vi "LDA_Maths_check.vi"(0 "B1 Close P11":dbl[](array[numeric])=[2570.8702, 433.495, 303.3539], 1 "Use Specification Beam Half-Angle":bool=TRUE, 5 "B1 Far P12":dbl[](array[numeric])=[2646.4891, 432.64, 306.6406], 7 "B2 Close P22":dbl[](array[numeric]), 9 "B2 Far P21":dbl[](array[numeric])=[2643.8249, 436.46, 319.8555], 11 "Use Green Beams (True) or Blue Beams (False)":bool, 12 "Beam Half-Angle (deg)":dbl=4.572782629722086 format="%#_9g", 13 "Using 45 Degree Mirror?":bool) -> (4 "Beam Data":T1={"Vg1 (Green 1 dir. vect.)"=[-0.9913846154927373, -0.08722653267640797, -0.09771425771896834], "Vg2  (Green 2 dir. vect.)"=[-0.987756229722306, 0.06610682889995216, -0.1413064677131501], "Vb1 (Blue 1 dir. vect.)"=[-0.9989930425665134, 0.011295311772511737, -0.04342023532481111], "Vb2 (Blue 1 dir. vect.)"=[-0.9801478026485297, -0.032415015548967537, -0.19560049010730732], "Porb (Orb XYZ posn. forced coplanar)"=[2558.4254936976226, 433.635708525098, 302.8130032638134], "Porb (Orb XYZ posn. - allow skew)"=[2558.425493697624, 433.635708525098, 302.8130032638134], "Orb posn. uncertainty, +/- dx, dy, dz"=[6.821210263296962e-13, 0.0, 0.0], "Vp (Actual Probe dir. vect)"=[-0.9927304194336236, -0.010593572680289348, -0.11989199535001965], "Yaw (deg)"=179.38861149501568, "Pitch (deg)"=-6.885869367545546, "In-Plane Roll (deg)"=15.984421506271559, "Beam Half Angle (deg)"=4.572782629722086, "B1 Close P11"=[2570.8702, 433.495, 303.3539], "B1 Far P12"=[2646.4891, 432.64, 306.6406], "B2 Close P22"=[nan, nan, nan], "B2 Far P21"=[2643.8249, 436.46, 319.8555], "Projected Roll (deg)"=15.87029035209838, "Green Velocity Vector"=[-0.022755515757454235, -0.9616341663360687, 0.273389679098803], "Blue Velocity Vector"=[0.1181884124343585, -0.2741304549899585, -0.9544024270784544], "Probe is facing...."="Upstream (YZ)", "Calculation Method"=""} {"Vp (Actual Probe dir. vect)" format="%#_6f"; "Vg2  (Green 2 dir. vect.)" format="%#_6f"; "Vg1 (Green 1 dir. vect.)" format="%#_6f"})   [LabVIEW 2011]
uses:
  Controls/LDA_Beam_Cluster.ctl
  <vilib>/Analysis/baseanly.llb/Unit Vector (DBL).vi
  <vilib>/Analysis/baseanly.llb/Real Dot Product.vi
  <vilib>/Analysis/NI_AALBase.lvlib
panel:
  # "Please note angle conventions:\nClockwise positive looking into the axis of rotation"
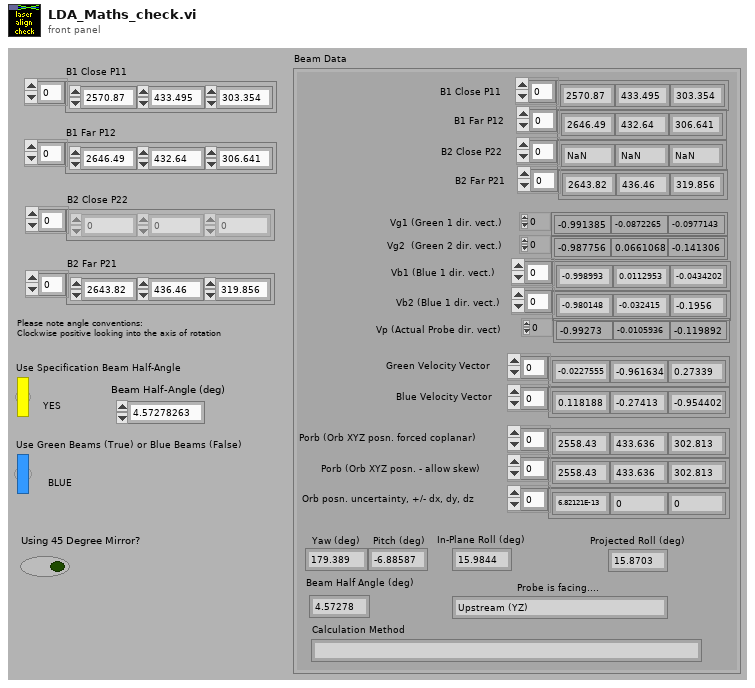
[diagram p1: front panel]
types:
  T1 = typedef "LDA_Beam_Cluster.ctl" = cluster{"Vg1 (Green 1 dir. vect.)":dbl[], "Vg2  (Green 2 dir. vect.)":dbl[], "Vb1 (Blue 1 dir. vect.)":dbl[], "Vb2 (Blue 1 dir. vect.)":dbl[], "Porb (Orb XYZ posn. forced coplanar)":dbl[], "Porb (Orb XYZ posn. - allow skew)":dbl[], "Orb posn. uncertainty, +/- dx, dy, dz":dbl[], "Vp (Actual Probe dir. vect)":dbl[], "Yaw (deg)":dbl, "Pitch (deg)":dbl, "In-Plane Roll (deg)":dbl, "Beam Half Angle (deg)":dbl, "B1 Close P11":dbl[], "B1 Far P12":dbl[], "B2 Close P22":dbl[], "B2 Far P21":dbl[], "Projected Roll (deg)":dbl, "Green Velocity Vector":dbl[], "Blue Velocity Vector":dbl[], "Probe is facing....":string, "Calculation Method":string}
  T2 = cluster{"Unit Vector[0]":dbl, "Unit Vector[1]":dbl, "Unit Vector[2]":dbl}
  T3 = cluster{"input variable":dbl, "input variable":dbl, "input variable":dbl}
  T4 = cluster{"input variable":dbl, dbl, "input variable":dbl}
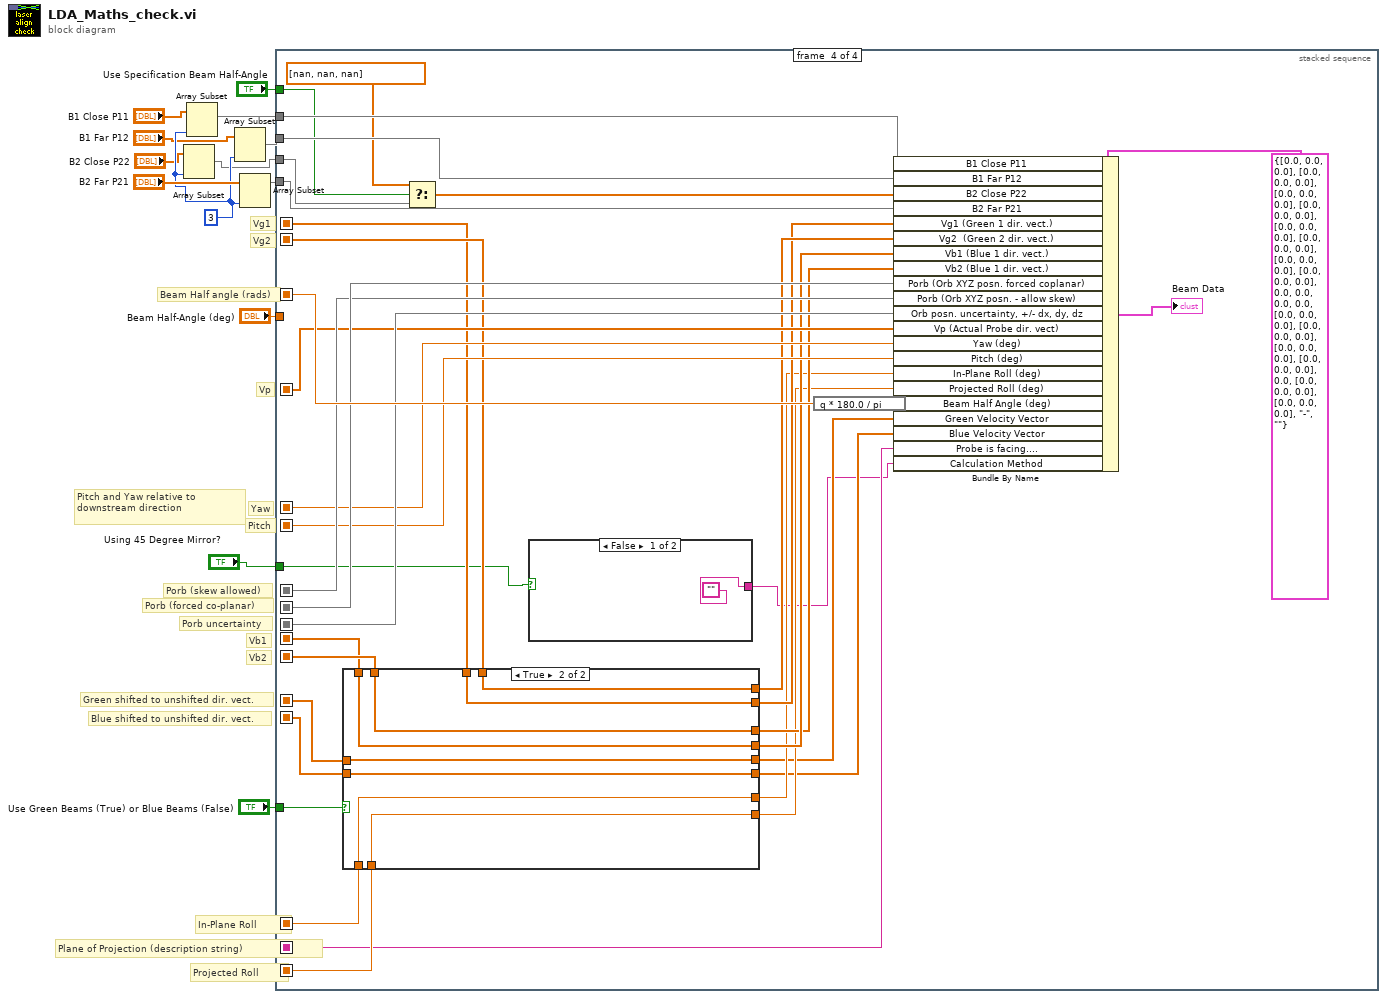
[diagram p0: block diagram]
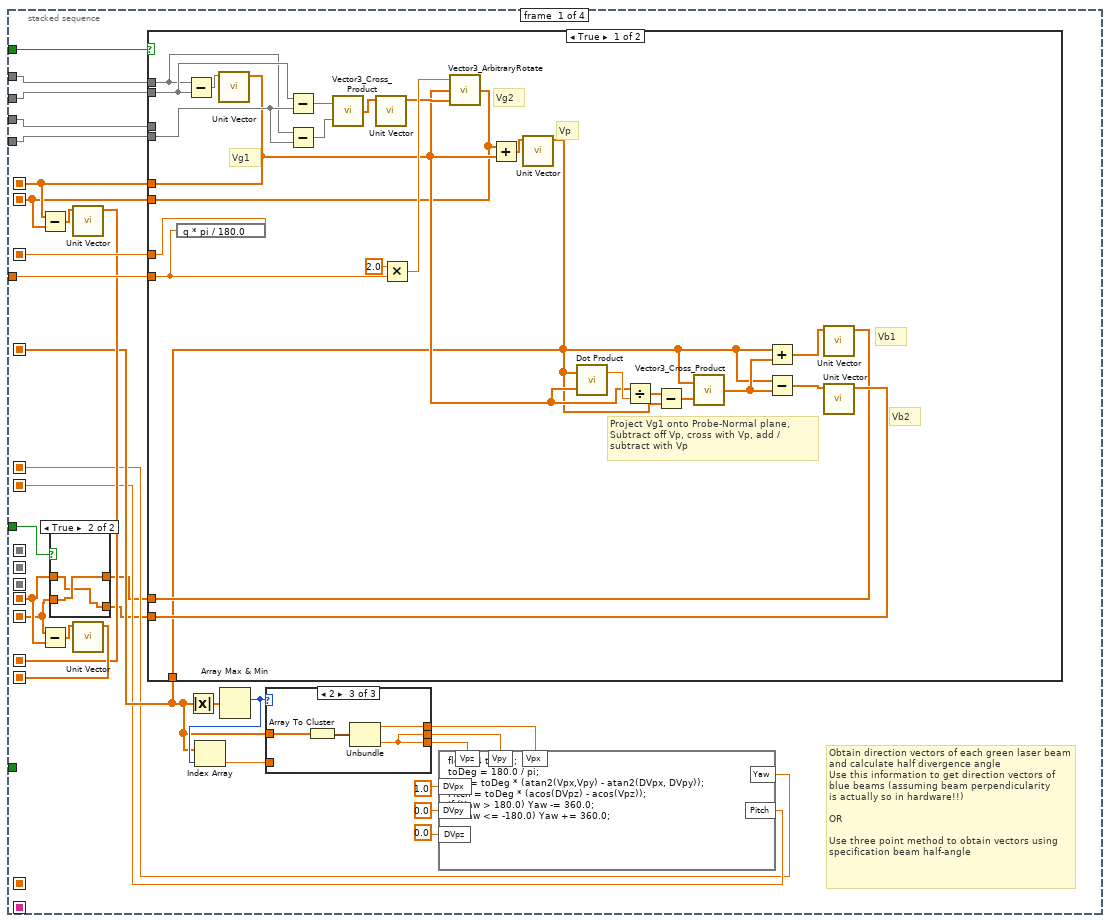
[diagram p2: hidden frame]
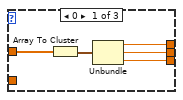
[diagram p4: hidden frame]
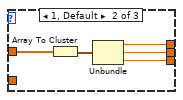
[diagram p5: hidden frame]
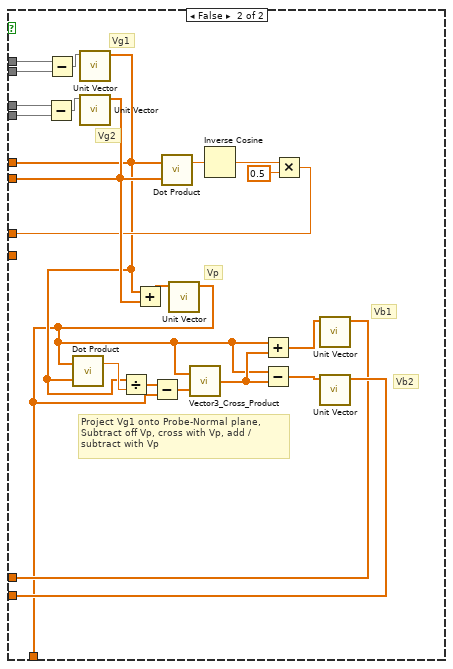
[diagram p6: hidden frame]
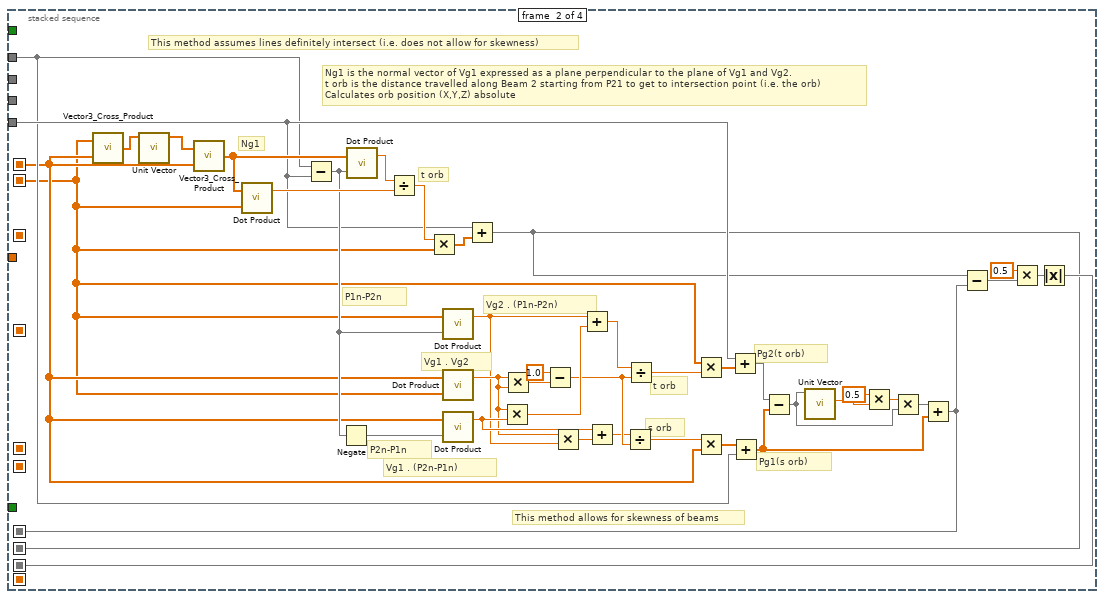
[diagram p7: hidden frame]
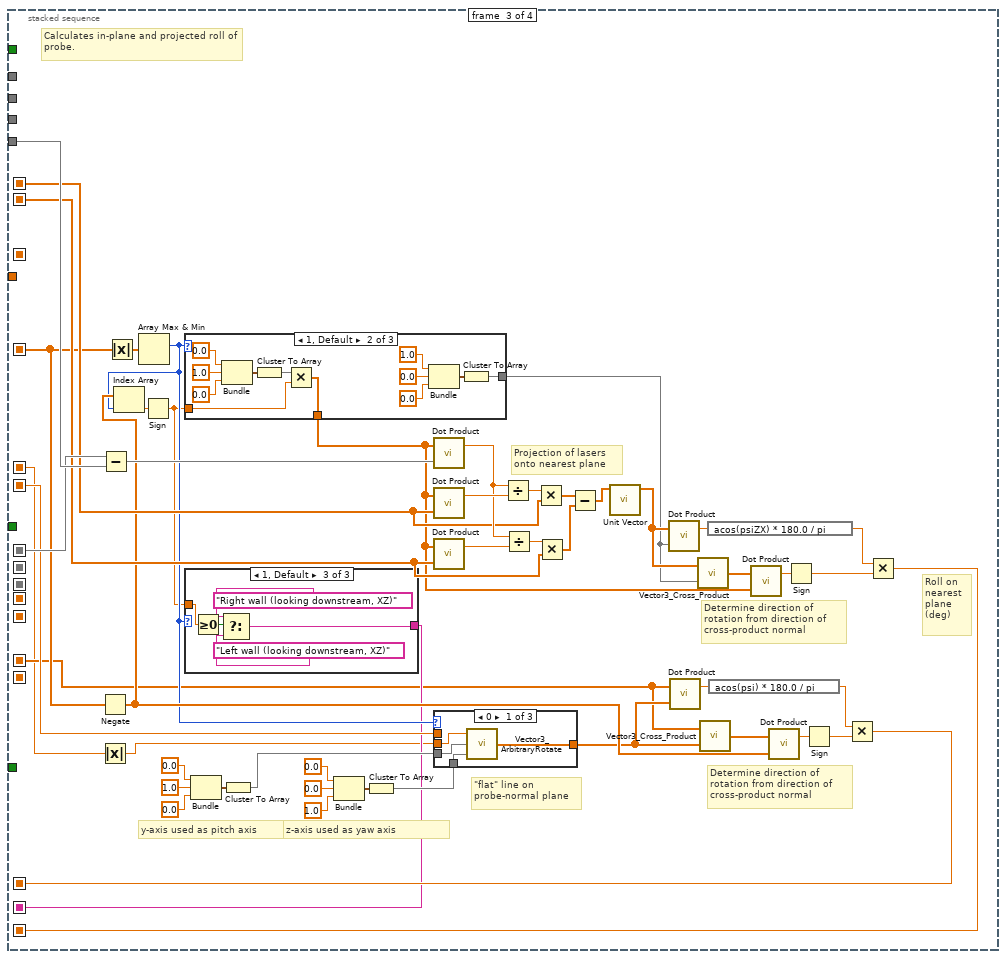
[diagram p8: hidden frame]
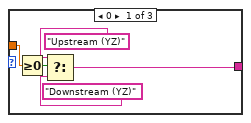
[diagram p9: hidden frame]
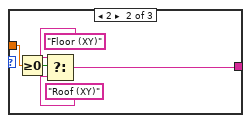
[diagram p10: hidden frame]
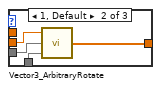
[diagram p11: hidden frame]
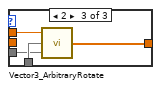
[diagram p12: hidden frame]
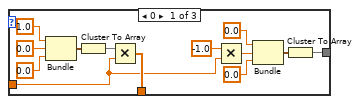
[diagram p13: hidden frame]
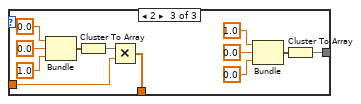
[diagram p14: hidden frame]
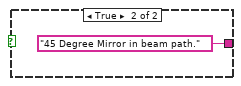
[diagram p15: hidden frame]
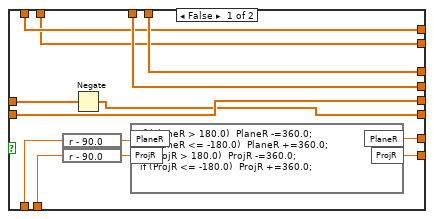
[diagram p16: hidden frame]
diagram:
  w5 = 3 ("length")
  # "Plane of Projection (description string)"
  # "Blue shifted to unshifted dir. vect."
  # "Green shifted to unshifted dir. vect."
  # "Projected Roll"
  # "Porb (forced co-planar)"
  # "Porb uncertainty"
  # "In-Plane Roll"
  # "Pitch"
  # "Yaw"
  # "Vb2"
  # "Vb1"
  # "Pitch and Yaw relative to\ndownstream direction"
  # "Vp"
  # "Porb (skew allowed)"
  # "Beam Half angle (rads)"
  # "Vg2"
  # "Vg1"
  n1 = Array Subset(array="B2 Close P22", length=w5) -> (w3:dbl[])  [unwired: 1 in]
  n2 = Array Subset(array="B1 Close P11", length=w5) -> (w6:dbl[])  [unwired: 1 in]
  n3 = Array Subset(array="B1 Far P12", length=w5) -> (w8:dbl[])  [unwired: 1 in]
  n4 = Array Subset(array="B2 Far P21", length=w5) -> (w9:dbl[])  [unwired: 1 in]
  n5 = stacked-sequence {
    seq-local: [w36 _ _ _] -> [_ w109 w171 w281]
    seq-local: [w35 _ _ _] -> [_ w108 w170 w282]
    seq-local: [w42 _ _ _] -> [_ _ _ w297]
    seq-local: [_ w112 _ _] -> [_ _ w177 w295]
    seq-local: [w24 _ _ _] -> [_ _ w162 w293]
    seq-local: [w17 _ _ _] -> [_ _ _ w279]
    seq-local: [w15 _ _ _] -> [_ _ _ w280]
    seq-local: [w19 _ _ _] -> [_ _ w150 w292]
    seq-local: [w20 _ _ _] -> [_ _ w176 w291]
    seq-local: [_ _ w179 _] -> [_ _ _ w273]
    seq-local: [_ w111 _ _] -> [_ _ _ w294]
    seq-local: [_ w110 _ _] -> [_ _ _ w296]
    seq-local: [_ _ w154 _] -> [_ _ _ w271]
    seq-local: [w31 _ _ _] -> [_ _ w151 w268]
    seq-local: [w33 _ _ _] -> [_ _ _ w269]
    seq-local: [_ _ w152 _] -> [_ _ _ w265]
    tunnel: w6 -> [w39 w123 _ w288]
    tunnel: w8 -> [w41 _ _ w289]
    tunnel: w3 -> [w43 _ _ w285]
    tunnel: w9 -> [w40 w128 w178 w290]
    tunnel: "Beam Half-Angle (deg)" -> [w38 _ _ _]
    tunnel: "Use Specification Beam Half-Angle" -> [w37 _ _ w286]
    tunnel: "Use Green Beams (True) or Blue Beams (False)" -> [_ _ _ w278]
    tunnel: "Using 45 Degree Mirror?" -> [w18 _ _ w263]
    frame #0 {
      # "Obtain direction vectors of each green laser beam and calculate half divergence angle\nUse this information to get direction vectors of blue beams (assuming beam perpendicularity\nis actually so in hardware!!)\n\nOR\n\nUse three point method to obtain vectors using specification beam half-angle"
      n6 = case shown="True" w37 {
        tunnel: w43 -> [_ w105]
        tunnel: [w67 w102] -> w35
        tunnel: [w64 w98] -> w42
        tunnel: [w66 w93] -> w14
        tunnel: w41 -> [w84 w92]
        tunnel: w40 -> [w83 w91]
        tunnel: w39 -> [w82 w90]
        tunnel: w38 -> [w63 _]
        tunnel: [w65 w89] -> w16
        tunnel: [w68 w87] -> w36
        tunnel: [w62 w86] -> w24
        frame True {
          # "Vg1"
          # "Vb2"
          # "Vb1"
          # "Vp"
          # "Vg2"
          # "Project Vg1 onto Probe-Normal plane, Subtract off Vp, cross with Vp, add / subtract with Vp"
          n7 = expression code="q * pi / 180.0"(w63) -> (w64:dbl)
          n8 = Subtract(x=w82, y=w84) -> (x-y=w85:dbl[])
          n9 = call-poly <vilib>:"Unit Vector.vi"("Input Vector"=w85) -> ("Unit Vector"=w68:dbl[])  [unwired: 2 in, 8 out]
          n10 = Subtract(x=w84, y=w83) -> (x-y=w81:dbl[])
          n11 = Subtract(x=w82, y=w83) -> (x-y=w80:dbl[])
          n12 = call "Vector3_Cross_Product.vi"("V"=w80, "U"=w81) -> ("UxV"=w79:dbl[])
          n13 = call-poly <vilib>:"Unit Vector.vi"("Input Vector"=w79) -> ("Unit Vector"=w76:dbl[])  [unwired: 2 in, 8 out]
          n14 = Multiply(x=2.0 ("y"), y=w63) -> (x*y=w77:dbl)
          n15 = call "Vector3_ArbitraryRotate.vi"("Arbitrary Axis (as UNIT Vector3)"=w76, "Input Vector3"=w68, "Rotation angle (deg)"=w77) -> ("Output Vector3"=w67:dbl[])
          n16 = Add(x=w67, y=w68) -> (x+y=w75:dbl[])
          n17 = call-poly <vilib>:"Unit Vector.vi"("Input Vector"=w75) -> ("Unit Vector"=w62:dbl[])  [unwired: 2 in, 8 out]
          n18 = call-poly <vilib>:"Dot Product.vi"("Y Vector"=w68, "X Vector"=w62) -> ("X * Y"=w70:dbl)  [unwired: 1 out]
          n19 = Divide(x=w68, y=w70) -> (x/y=w71:dbl[])
          n20 = Subtract(x=w71, y=w62) -> (x-y=w72:dbl[])
          n21 = call "Vector3_Cross_Product.vi"("V"=w72, "U"=w62) -> ("UxV"=w73:dbl[])
          n22 = Add(x=w62, y=w73) -> (x+y=w74:dbl[])
          n23 = Subtract(x=w62, y=w73) -> (x-y=w69:dbl[])
          n24 = call-poly <vilib>:"Unit Vector.vi"("Input Vector"=w74) -> ("Unit Vector"=w65:dbl[])  [unwired: 2 in, 8 out]
          n25 = call-poly <vilib>:"Unit Vector.vi"("Input Vector"=w69) -> ("Unit Vector"=w66:dbl[])  [unwired: 2 in, 8 out]
        }
        frame False {
          # "Vg2"
          # "Vg1"
          # "Vb2"
          # "Vb1"
          # "Vp"
          # "Project Vg1 onto Probe-Normal plane, Subtract off Vp, cross with Vp, add / subtract with Vp"
          n26 = Subtract(x=w105, y=w91) -> (x-y=w106:dbl[])
          n27 = Subtract(x=w90, y=w92) -> (x-y=w107:dbl[])
          n28 = call-poly <vilib>:"Unit Vector.vi"("Input Vector"=w107) -> ("Unit Vector"=w87:dbl[])  [unwired: 2 in, 8 out]
          n29 = call-poly <vilib>:"Unit Vector.vi"("Input Vector"=w106) -> ("Unit Vector"=w102:dbl[])  [unwired: 2 in, 8 out]
          n30 = Add(x=w87, y=w102) -> (x+y=w101:dbl[])
          n31 = call-poly <vilib>:"Dot Product.vi"("Y Vector"=w102, "X Vector"=w87) -> ("X * Y"=w100:dbl)  [unwired: 1 out]
          n32 = call-poly <vilib>:"Unit Vector.vi"("Input Vector"=w101) -> ("Unit Vector"=w86:dbl[])  [unwired: 2 in, 8 out]
          n33 = call-poly <vilib>:"Dot Product.vi"("Y Vector"=w87, "X Vector"=w86) -> ("X * Y"=w97:dbl)  [unwired: 1 out]
          n34 = Divide(x=w87, y=w97) -> (x/y=w96:dbl[])
          n35 = Subtract(x=w96, y=w86) -> (x-y=w95:dbl[])
          n36 = call "Vector3_Cross_Product.vi"("V"=w95, "U"=w86) -> ("UxV"=w94:dbl[])
          n37 = Inverse Cosine(1:w100) -> (0:w104:dbl)
          n38 = Add(x=w86, y=w94) -> (x+y=w88:dbl[])
          n39 = Subtract(x=w86, y=w94) -> (x-y=w99:dbl[])
          n40 = Multiply(x=w104, y=0.5) -> (x*y=w98:dbl)
          n41 = call-poly <vilib>:"Unit Vector.vi"("Input Vector"=w88) -> ("Unit Vector"=w89:dbl[])  [unwired: 2 in, 8 out]
          n42 = call-poly <vilib>:"Unit Vector.vi"("Input Vector"=w99) -> ("Unit Vector"=w93:dbl[])  [unwired: 2 in, 8 out]
        }
      }
      n43 = Subtract(x=w36, y=w35) -> (x-y=w32:dbl[])
      n44 = case shown="True" w18 {
        tunnel: [w45 w46] -> w17
        tunnel: w16 -> [w45 w47]
        tunnel: [w44 w47] -> w15
        tunnel: w14 -> [w44 w46]
        frame False {
        }
        frame True {
        }
      }
      n45 = Subtract(x=w15, y=w17) -> (x-y=w34:dbl[])
      n46 = call-poly <vilib>:"Unit Vector.vi"("Input Vector"=w32) -> ("Unit Vector"=w31:dbl[])  [unwired: 2 in, 8 out]
      n47 = call-poly <vilib>:"Unit Vector.vi"("Input Vector"=w34) -> ("Unit Vector"=w33:dbl[])  [unwired: 2 in, 8 out]
      n48 = Absolute Value(x=w24) -> (abs(x)=w30:dbl[])
      n49 = Array Max & Min(array=w30) -> (max index (indices)=w29:i32)  [unwired: 3 out]
      n50 = Index Array(array=w24, index=w29) -> (element=w25:dbl)
      n51 = case shown="2" w29 {
        tunnel: w25 -> [_ _ _]
        tunnel: w24 -> [w51 w56 w60]
        tunnel: [w50 w53 w59] -> w21
        tunnel: [w49 w54 w59] -> w22
        tunnel: [w48 w55 w58] -> w23
        frame 0 {
          n52 = Array To Cluster(array=w51) -> (cluster=w52:T2)
          n53 = Unbundle(w52) -> ("Unit Vector[0]"=w48:dbl, "Unit Vector[1]"=w49:dbl, "Unit Vector[2]"=w50:dbl)
        }
        frame 1, Default {
          n54 = Array To Cluster(array=w56) -> (cluster=w57:T2)
          n55 = Unbundle(w57) -> ("Unit Vector[0]"=w55:dbl, "Unit Vector[1]"=w54:dbl, "Unit Vector[2]"=w53:dbl)
        }
        frame 2 {
          n56 = Array To Cluster(array=w60) -> (cluster=w61:T2)
          n57 = Unbundle(w61) -> ("Unit Vector[0]"=w58:dbl, "Unit Vector[2]"=w59:dbl)  [unwired: 1 out]
        }
      }
      n58 = formula code="float64 toDeg;\ntoDeg = 180.0 / pi;\nYaw = toDeg * (atan2(Vpx,Vpy) - atan2(DVpx, DVpy));\nPitch = toDeg * (acos(DVpz) - acos(Vpz));\nif (Yaw > 180.0) Yaw -= 360.0;\nif (Yaw <= -180.0) Yaw += 360.0;"("Vpx"=w23, "Vpy"=w22, "Vpz"=w21, "DVpx"=1.0 ("input variable"), "DVpy"=0.0 ("input variable"), "DVpz"=0.0 ("input variable")) -> ("Yaw"=w19:dbl, "Pitch"=w20:dbl)
    }
    frame #1 {
      # "Pg1(s orb)"
      # "Pg2(t orb)"
      # "s orb"
      # "t orb"
      # "Vg1 . (P2n-P1n)"
      # "Vg1 . Vg2"
      # "Vg2 . (P1n-P2n)"
      # "P2n-P1n"
      # "P1n-P2n"
      # "This method allows for skewness of beams"
      # "This method assumes lines definitely intersect (i.e. does not allow for skewness)"
      # "t orb"
      # "Ng1 is the normal vector of Vg1 expressed as a plane perpendicular to the plane of Vg1 and Vg2.\nt orb is the distance travelled along Beam 2 starting from P21 to get to intersection point (i.e. the orb)\nCalculates orb position (X,Y,Z) absolute"
      # "Ng1"
      n59 = call "Vector3_Cross_Product.vi"("V"=w109, "U"=w108) -> ("UxV"=w143:dbl[])
      n60 = call-poly <vilib>:"Unit Vector.vi"("Input Vector"=w143) -> ("Unit Vector"=w142:dbl[])  [unwired: 2 in, 8 out]
      n61 = call "Vector3_Cross_Product.vi"("V"=w109, "U"=w142) -> ("UxV"=w141:dbl[])
      n62 = call-poly <vilib>:"Dot Product.vi"("Y Vector"=w108, "X Vector"=w141) -> ("X * Y"=w146:dbl)  [unwired: 1 out]
      n63 = Subtract(x=w123, y=w128) -> (x-y=w140:dbl[])
      n64 = Negate(x=w140) -> (-x=w139:dbl[])
      n65 = call-poly <vilib>:"Dot Product.vi"("Y Vector"=w140, "X Vector"=w141) -> ("X * Y"=w147:dbl)  [unwired: 1 out]
      n66 = Divide(x=w147, y=w146) -> (x/y=w145:dbl)
      n67 = Multiply(x=w145, y=w108) -> (x*y=w144:dbl[])
      n68 = call-poly <vilib>:"Dot Product.vi"("Y Vector"=w140, "X Vector"=w108) -> ("X * Y"=w132:dbl)  [unwired: 1 out]
      n69 = call-poly <vilib>:"Dot Product.vi"("Y Vector"=w108, "X Vector"=w109) -> ("X * Y"=w133:dbl)  [unwired: 1 out]
      n70 = call-poly <vilib>:"Dot Product.vi"("Y Vector"=w139, "X Vector"=w109) -> ("X * Y"=w134:dbl)  [unwired: 1 out]
      n71 = Add(x=w128, y=w144) -> (x+y=w110:dbl[])
      n72 = Multiply(x=w133, y=w134) -> (x*y=w136:dbl)
      n73 = Multiply(x=w133, y=w133) -> (x*y=w137:dbl)
      n74 = Subtract(x=1.0, y=w137) -> (x-y=w130:dbl)
      n75 = Multiply(x=w133, y=w132) -> (x*y=w131:dbl)
      n76 = Add(x=w132, y=w136) -> (x+y=w135:dbl)
      n77 = Add(x=w134, y=w131) -> (x+y=w129:dbl)
      n78 = Divide(x=w129, y=w130) -> (x/y=w125:dbl)
      n79 = Divide(x=w135, y=w130) -> (x/y=w127:dbl)
      n80 = Multiply(x=w108, y=w127) -> (x*y=w126:dbl[])
      n81 = Multiply(x=w125, y=w109) -> (x*y=w124:dbl[])
      n82 = Add(x=w128, y=w126) -> (x+y=w122:dbl[])
      n83 = Add(x=w124, y=w123) -> (x+y=w116:dbl[])
      n84 = Subtract(x=w122, y=w116) -> (x-y=w118:dbl[])
      n85 = call-poly <vilib>:"Unit Vector.vi"("Input Vector"=w118) -> ("norm"=w120:dbl)  [unwired: 2 in, 8 out]
      n86 = Multiply(x=0.5, y=w120) -> (x*y=w119:dbl)
      n87 = Multiply(x=w119, y=w118) -> (x*y=w117:dbl[])
      n88 = Add(x=w117, y=w116) -> (x+y=w112:dbl[])
      n89 = Subtract(x=w110, y=w112) -> (x-y=w114:dbl[])
      n90 = Multiply(x=0.5, y=w114) -> (x*y=w113:dbl[])
      n91 = Absolute Value(x=w113) -> (abs(x)=w111:dbl[])
    }
    frame #2 {
      # "y-axis used as pitch axis"
      # "z-axis used as yaw axis"
      # "Roll on nearest plane (deg)"
      # "Determine direction of rotation from direction of cross-product normal"
      # "\"flat\" line on probe-normal plane"
      # "Determine direction of rotation from direction of cross-product normal"
      # "Projection of lasers onto nearest plane"
      # "Calculates in-plane and projected roll of probe."
      n92 = Negate(x=w162) -> (-x=w161:dbl[])
      n93 = Absolute Value(x=w150) -> (abs(x)=w149:dbl)
      n94 = Subtract(x=w177, y=w178) -> (x-y=w197:dbl[])
      n95 = Absolute Value(x=w162) -> (abs(x)=w168:dbl[])
      n96 = Array Max & Min(array=w168) -> (max index (indices)=w153:i32)  [unwired: 3 out]
      n97 = Index Array(array=w161, index=w153) -> (element=w169:dbl)
      n98 = Sign(1:w169) -> (0:w148:dbl)
      n99 = case shown="1, Default" w153 {
        tunnel: [w229 w240 w250] -> w160
        tunnel: w148 -> [w227 w238 w257]
        tunnel: [w228 w239 w251] -> w155
        frame 0 {
          n100 = Bundle("input variable"=1.0, "input variable"=0.0, "input variable"=0.0) -> (w234:T3)  [unwired: 1 out]
          n101 = Cluster To Array(cluster=w234) -> (array=w233:dbl[])
          n102 = Multiply(x=w233, y=w227) -> (x*y=w229:dbl[])
          n103 = Multiply(x=-1.0 ("input variable"), y=w227) -> (x*y=w226:dbl)
          n104 = Bundle("input variable"=0.0, w226, "input variable"=0.0) -> (w230:T4)  [unwired: 1 out]
          n105 = Cluster To Array(cluster=w230) -> (array=w228:dbl[])
        }
        frame 1, Default {
          n106 = Bundle("input variable"=0.0, "input variable"=1.0, "input variable"=0.0) -> (w246:T3)  [unwired: 1 out]
          n107 = Cluster To Array(cluster=w246) -> (array=w245:dbl[])
          n108 = Multiply(x=w245, y=w238) -> (x*y=w240:dbl[])
          n109 = Bundle("input variable"=1.0, "input variable"=0.0, "input variable"=0.0) -> (w241:T3)  [unwired: 1 out]
          n110 = Cluster To Array(cluster=w241) -> (array=w239:dbl[])
        }
        frame 2 {
          n111 = Bundle("input variable"=0.0, "input variable"=0.0, "input variable"=1.0) -> (w258:T3)  [unwired: 1 out]
          n112 = Cluster To Array(cluster=w258) -> (array=w256:dbl[])
          n113 = Multiply(x=w256, y=w257) -> (x*y=w250:dbl[])
          n114 = Bundle("input variable"=1.0, "input variable"=0.0, "input variable"=0.0) -> (w252:T3)  [unwired: 1 out]
          n115 = Cluster To Array(cluster=w252) -> (array=w251:dbl[])
        }
      }
      n116 = case shown="1, Default" w153 {
        tunnel: w148 -> [w202 w207 w212]
        tunnel: [w198 w203 w208] -> w152
        frame 0 {
          n117 = Greater Or Equal To 0?(x=w202) -> (x >= 0?=w201:bool)
          n118 = Select(t="Upstream (YZ)", s=w201, f="Downstream (YZ)") -> (s? t:f=w198:string)
        }
        frame 2 {
          n119 = Greater Or Equal To 0?(x=w207) -> (x >= 0?=w206:bool)
          n120 = Select(t="Floor (XY)", s=w206, f="Roof (XY)") -> (s? t:f=w203:string)
        }
        frame 1, Default {
          n121 = Greater Or Equal To 0?(x=w212) -> (x >= 0?=w211:bool)
          n122 = Select(t="Right wall (looking downstream, XZ)", s=w211, f="Left wall (looking downstream, XZ)") -> (s? t:f=w208:string)
        }
      }
      n123 = Bundle("input variable"=0.0, "input variable"=1.0, "input variable"=0.0) -> (w175:T3)  [unwired: 1 out]
      n124 = Cluster To Array(cluster=w175) -> (array=w158:dbl[])
      n125 = Bundle("input variable"=0.0, "input variable"=0.0, "input variable"=1.0) -> (w167:T3)  [unwired: 1 out]
      n126 = Cluster To Array(cluster=w167) -> (array=w159:dbl[])
      n127 = call-poly <vilib>:"Dot Product.vi"("Y Vector"=w197, "X Vector"=w160) -> ("X * Y"=w194:dbl)  [unwired: 1 out]
      n128 = call-poly <vilib>:"Dot Product.vi"("Y Vector"=w171, "X Vector"=w160) -> ("X * Y"=w196:dbl)  [unwired: 1 out]
      n129 = call-poly <vilib>:"Dot Product.vi"("Y Vector"=w170, "X Vector"=w160) -> ("X * Y"=w193:dbl)  [unwired: 1 out]
      n130 = case shown="0" w153 {
        tunnel: w159 -> [w214 w220 w222]
        tunnel: w176 -> [_ _ w224]
        tunnel: [w213 w217 w223] -> w157
        tunnel: w158 -> [w215 w219 w221]
        tunnel: w149 -> [w216 w218 _]
        frame 0 {
          n131 = call "Vector3_ArbitraryRotate.vi"("Arbitrary Axis (as UNIT Vector3)"=w214, "Input Vector3"=w215, "Rotation angle (deg)"=w216) -> ("Output Vector3"=w213:dbl[])
        }
        frame 1, Default {
          n132 = call "Vector3_ArbitraryRotate.vi"("Arbitrary Axis (as UNIT Vector3)"=w220, "Input Vector3"=w219, "Rotation angle (deg)"=w218) -> ("Output Vector3"=w217:dbl[])
        }
        frame 2 {
          n133 = call "Vector3_ArbitraryRotate.vi"("Arbitrary Axis (as UNIT Vector3)"=w221, "Input Vector3"=w222, "Rotation angle (deg)"=w224) -> ("Output Vector3"=w223:dbl[])
        }
      }
      n134 = Divide(x=w194, y=w196) -> (x/y=w195:dbl)
      n135 = Divide(x=w194, y=w193) -> (x/y=w192:dbl)
      n136 = Multiply(x=w195, y=w171) -> (x*y=w188:dbl[])
      n137 = Multiply(x=w192, y=w170) -> (x*y=w187:dbl[])
      n138 = Subtract(x=w188, y=w187) -> (x-y=w190:dbl[])
      n139 = call-poly <vilib>:"Unit Vector.vi"("Input Vector"=w190) -> ("Unit Vector"=w156:dbl[])  [unwired: 2 in, 8 out]
      n140 = call-poly <vilib>:"Dot Product.vi"("Y Vector"=w155, "X Vector"=w156) -> ("X * Y"=w191:dbl)  [unwired: 1 out]
      n141 = call-poly <vilib>:"Dot Product.vi"("Y Vector"=w157, "X Vector"=w151) -> ("X * Y"=w189:dbl)  [unwired: 1 out]
      n142 = call "Vector3_Cross_Product.vi"("V"=w155, "U"=w156) -> ("UxV"=w181:dbl[])
      n143 = call "Vector3_Cross_Product.vi"("V"=w157, "U"=w151) -> ("UxV"=w186:dbl[])
      n144 = expression code="acos(psiZX) * 180.0 / pi"(w191) -> (w180:dbl)
      n145 = expression code="acos(psi) * 180.0 / pi"(w189) -> (w184:dbl)
      n146 = call-poly <vilib>:"Dot Product.vi"("Y Vector"=w160, "X Vector"=w181) -> ("X * Y"=w182:dbl)  [unwired: 1 out]
      n147 = call-poly <vilib>:"Dot Product.vi"("Y Vector"=w161, "X Vector"=w186) -> ("X * Y"=w185:dbl)  [unwired: 1 out]
      n148 = Sign(1:w182) -> (0:w163:dbl)
      n149 = Sign(1:w185) -> (0:w183:dbl)
      n150 = Multiply(x=w184, y=w183) -> (x*y=w179:dbl)
      n151 = Multiply(x=w180, y=w163) -> (x*y=w154:dbl)
    }
    frame #3 {
      n152 = case shown="True" w278 {
        tunnel: w282 -> [w312 w320]
        tunnel: w281 -> [w313 w321]
        tunnel: w280 -> [w310 w318]
        tunnel: w279 -> [w311 w319]
        tunnel: [w310 w321] -> w276
        tunnel: [w311 w320] -> w277
        tunnel: [w313 w319] -> w275
        tunnel: [w312 w318] -> w274
        tunnel: w273 -> [w308 w317]
        tunnel: w271 -> [w309 w316]
        tunnel: [w304 w317] -> w272
        tunnel: [w303 w316] -> w270
        tunnel: w269 -> [w307 w314]
        tunnel: w268 -> [w302 w315]
        tunnel: [w307 w315] -> w266
        tunnel: [w301 w314] -> w267
        frame False {
          n153 = expression code="r - 90.0"(w308) -> (w306:dbl)
          n154 = expression code="r - 90.0"(w309) -> (w305:dbl)
          n155 = Negate(x=w302) -> (-x=w301:dbl[])
          n156 = formula code="if (PlaneR > 180.0)  PlaneR -=360.0;\nif (PlaneR <= -180.0)  PlaneR +=360.0;\nif (ProjR > 180.0)  ProjR -=360.0;\nif (ProjR <= -180.0)  ProjR +=360.0;"("PlaneR"=w306, "ProjR"=w305) -> ("PlaneR"=w304:dbl, "ProjR"=w303:dbl)
        }
        frame True {
        }
      }
      n157 = Select(t=dbl[] [nan, nan, nan], s=w286, f=w285) -> (s? t:f=w284:dbl[])
      n158 = case shown="False" w263 {
        tunnel: ["" "45 Degree Mirror in beam path."] -> w262
        frame False {
        }
        frame True {
        }
      }
      n159 = expression code="q * 180.0 / pi"(w297) -> (w287:dbl)
      n160 = Bundle By Name(cluster=T1 {"Vg1 (Green 1 dir. vect.)"=[0.0, 0.0, 0.0], "Vg2  (Green 2 dir. vect.)"=[0.0, 0.0, 0.0], "Vb1 (Blue 1 dir. vect.)"=[0.0, 0.0, 0.0], "Vb2 (Blue 1 dir. vect.)"=[0.0, 0.0, 0.0], "Porb (Orb XYZ posn. forced coplanar)"=[0.0, 0.0, 0.0], "Porb (Orb XYZ posn. - allow skew)"=[0.0, 0.0, 0.0], "Orb posn. uncertainty, +/- dx, dy, dz"=[0.0, 0.0, 0.0], "Vp (Actual Probe dir. vect)"=[0.0, 0.0, 0.0], "Yaw (deg)"=0.0, "Pitch (deg)"=0.0, "In-Plane Roll (deg)"=0.0, "Beam Half Angle (deg)"=0.0, "B1 Close P11"=[0.0, 0.0, 0.0], "B1 Far P12"=[0.0, 0.0, 0.0], "B2 Close P22"=[0.0, 0.0, 0.0], "B2 Far P21"=[0.0, 0.0, 0.0], "Projected Roll (deg)"=0.0, "Green Velocity Vector"=[0.0, 0.0, 0.0], "Blue Velocity Vector"=[0.0, 0.0, 0.0], "Probe is facing...."="-", "Calculation Method"=""} ("input cluster"), "B1 Close P11"=w288, "B1 Far P12"=w289, "B2 Close P22"=w284, "B2 Far P21"=w290, "Vg1 (Green 1 dir. vect.)"=w276, "Vg2  (Green 2 dir. vect.)"=w277, "Vb1 (Blue 1 dir. vect.)"=w275, "Vb2 (Blue 1 dir. vect.)"=w274, "Porb (Orb XYZ posn. forced coplanar)"=w296, "Porb (Orb XYZ posn. - allow skew)"=w295, "Orb posn. uncertainty, +/- dx, dy, dz"=w294, "Vp (Actual Probe dir. vect)"=w293, "Yaw (deg)"=w292, "Pitch (deg)"=w291, "In-Plane Roll (deg)"=w272, "Projected Roll (deg)"=w270, "Beam Half Angle (deg)"=w287, "Green Velocity Vector"=w266, "Blue Velocity Vector"=w267, "Probe is facing...."=w265, "Calculation Method"=w262) -> (→"Beam Data":T1)
    }
  }
